vi "NMRvmeCard3.vi"() -> ()   [LabVIEW 2013]
uses:
  <vilib>/Utility/file.llb/Read From Spreadsheet File (DBL).vi
  <vilib>/Analysis/NI_AALBase.lvlib
panel:
  in  "Max":bool=TRUE
  in  "Logoffset (V)":dbl=-5.924000000000002 min=-9.0 max=0.0 step=0.0005 format="%_5g"
  in  "Phase (V)":dbl=6.5 min=0.0 max=9.0 step=0.0005 format="%_5g"
  out "Telnet error out":errorcluster
  in  "Real/Quad Q curve":bool=TRUE
  out "Temperature (C)":dbl(graph)=27.5
  out "+3V supply":dbl=3.245 format="%_4g"
  out "Temp (C)":dbl=27.5 format="%_4g"
  in  "RemovePed":bool=TRUE
  in  "IF / LOG Det":bool
  in  "Q curve file":string="realback213.txt"
  out "File name 2":string="C:\\users\\plm\\Desktop\\rssmt\\realback213.txt"
  in  "AutoTune":bool=TRUE
  out "RF OK":bool=TRUE
  out "Peak area (V-MHz)":sgl=0.028832752 format="%.5f"
  in  "Gauss Fit":bool
  out "NMR Graph + Fit":cluster{cluster{dbl, "Numeric":dbl}[]}[](graph)=[{[{212.6, "Numeric"=-0.048532500000002754}, {212.60999999999999, "Numeric"=-0.03653250000002278}, {212.62, "Numeric"=-0.045792499999980585}, {212.63, "Numeric"=-0.04201250000000012}, {212.64, "Numeric"=-0.04119250000001873}, {212.65, "Numeric"=-0.031632499999979746}, {212.66, "Numeric"=-0.02963249999999795}, {212.67, "Numeric"=-0.03309250000001501}, {212.68, "Numeric"=-0.02891249999997941}, {212.69, "Numeric"=-0.03189249999999605}, {212.7, "Numeric"=-0.022732500000011698}, {212.71, "Numeric"=-0.01753249999997938}, {212.72, "Numeric"=-0.024692499999994646}, {212.73, "Numeric"=-0.01491250000000879}, {212.74, "Numeric"=-0.010992500000022023}, {212.75, "Numeric"=-0.011032499999993586}, {212.76, "Numeric"=0.0010674999999937297}, {212.77, "Numeric"=-0.008192500000018001}, {212.78, "Numeric"=-0.02261249999999287}, {212.79, "Numeric"=-0.024392500000004116}, {212.8, "Numeric"=-0.032232500000014375}, {212.81, "Numeric"=-0.027532499999992573}, {212.82, "Numeric"=-0.02899250000000236}, {212.82999999999998, "Numeric"=-0.024212500000011152}, {212.84, "Numeric"=-0.03769249999999266}, {212.85, "Numeric"=-0.039132500000000986}, {212.85999999999999, "Numeric"=-0.023232500000008306}, {212.87, "Numeric"=-0.016892499999993125}, {212.88, "Numeric"=0.0014875000000000131}, {212.89, "Numeric"=-0.004392500000005847}, {212.9, "Numeric"=0.00376750000000603}, {212.91, "Numeric"=0.008167500000000622}, {212.92, "Numeric"=-0.00019250000000377299}, {212.93, "Numeric"=0.00618750000000479}, {212.94, "Numeric"=0.01090750000000085}, {212.95, "Numeric"=0.03826749999999793}, {212.96, "Numeric"=0.09656750000000316}, {212.97, "Numeric"=0.1705075000000007}, {212.98, "Numeric"=0.3255874999999992}, {212.99, "Numeric"=0.3123074999999988}, {213.0, "Numeric"=0.22976750000000018}, {213.01, "Numeric"=0.20266750000000014}, {213.02, "Numeric"=0.18930750000000116}, {213.03, "Numeric"=0.14968749999999922}, {213.04, "Numeric"=0.1382075000000007}, {213.05, "Numeric"=0.14966750000000317}, {213.06, "Numeric"=0.1471674999999979}, {213.07, "Numeric"=0.16360750000000085}, {213.08, "Numeric"=0.1525875000000048}, {213.09, "Numeric"=0.09930749999999622}, {213.1, "Numeric"=0.06516750000000061}, {213.11, "Numeric"=0.04746750000000602}, {213.12, "Numeric"=0.04960749999999414}, {213.13, "Numeric"=0.0405875}, {213.14000000000001, "Numeric"=0.024907500000006872}, {213.15, "Numeric"=0.013367499999991695}, {213.16, "Numeric"=0.014667499999999018}, {213.17000000000002, "Numeric"=0.029707500000007343}, {213.18, "Numeric"=0.04208749999998884}, {213.19, "Numeric"=0.029407499999997647}, {213.2, "Numeric"=0.038467500000007426}, {213.21, "Numeric"=0.038667499999985616}, {213.22, "Numeric"=0.016007499999995876}, {213.23, "Numeric"=0.023787500000007126}, {213.24, "Numeric"=0.03210750000001941}, {213.25, "Numeric"=0.03386749999999372}, {213.26, "Numeric"=0.015167500000006415}, {213.27, "Numeric"=0.018307500000020214}, {213.28, "Numeric"=0.0113874999999912}, {213.29, "Numeric"=0.021007500000005373}, {213.3, "Numeric"=0.0360675000000206}, {213.31, "Numeric"=0.03156749999998826}, {213.32, "Numeric"=0.03200750000000396}, {213.33, "Numeric"=0.0359875000000206}, {213.34, "Numeric"=0.032307499999984945}, {213.35, "Numeric"=0.03296750000000209}, {213.36, "Numeric"=0.026367500000020253}, {213.37, "Numeric"=0.016907499999981316}, {213.38, "Numeric"=0.011387499999999887}, {213.39000000000001, "Numeric"=0.014307500000019461}, {213.4, "Numeric"=0.018367499999977225}]}]
  in  "Amp of Q curve":dbl=2.800000000000001 min=0.0 max=9.0 step=0.01 format="%_3f"
  in  "Subtract Q curve":bool=TRUE
  in  "Adjust Tune":bool=TRUE
  out "Pedestal Offset":dbl(graph)=0.026662499999999974
  out "Pedestal Difference":dbl(graph)=0.05318500000000375
  out "# Good Spectra":i32=9865
  in  "Quality cuts":bool=TRUE
  out "Pedestal OK":bool=TRUE
  out "Sweep #":i32=122
  out "1st Sweep":bool
  out "ADC volts OK":bool=TRUE
  out "Peak Height Distribution":cluster{"Y":dbl[], "Y":dbl[]}[](graph)=[{"Y"=[0.29554139583333255, 0.2962908541666659, 0.29704031249999924, 0.2977897708333326, 0.2985392291666659, 0.29928868749999926, 0.3000381458333326, 0.3007876041666659, 0.30153706249999923, 0.3022865208333326, 0.3030359791666659, 0.30378543749999926, 0.3045348958333326, 0.3052843541666659, 0.3060338124999992, 0.30678327083333257, 0.3075327291666659, 0.30828218749999925, 0.3090316458333326, 0.30978110416666593, 0.3105305624999992, 0.31128002083333256, 0.3120294791666659, 0.31277893749999924, 0.3135283958333326, 0.3142778541666659, 0.31502731249999927, 0.31577677083333255, 0.3165262291666659, 0.31727568749999924, 0.3180251458333326, 0.3187746041666659, 0.31952406249999926, 0.32027352083333255, 0.3210229791666659, 0.32177243749999923, 0.3225218958333326, 0.3232713541666659, 0.32402081249999926, 0.3247702708333326, 0.3255197291666659, 0.3262691874999992, 0.32701864583333257, 0.3277681041666659, 0.32851756249999925, 0.3292670208333326, 0.33001647916666593, 0.3307659374999992, 0.33151539583333256, 0.3322648541666659, 0.33301431249999924, 0.3337637708333326, 0.3345132291666659, 0.3352626874999992, 0.33601214583333255, 0.3367616041666659, 0.33751106249999924, 0.3382605208333326, 0.3390099791666659, 0.33975943749999926, 0.34050889583333255, 0.3412583541666659, 0.34200781249999923, 0.3427572708333326, 0.3435067291666659, 0.34425618749999926, 0.3450056458333326, 0.3457551041666659, 0.3465045624999992, 0.34725402083333257, 0.3480034791666659, 0.34875293749999925, 0.3495023958333326, 0.3502518541666659, 0.3510013124999992, 0.35175077083333256, 0.3525002291666659, 0.35324968749999924, 0.3539991458333326, 0.3547486041666659, 0.3554980624999992, 0.35624752083333255, 0.3569969791666659, 0.35774643749999924, 0.3584958958333326, 0.3592453541666659, 0.35999481249999926, 0.36074427083333255, 0.3614937291666659, 0.36224318749999923, 0.3629926458333326, 0.3637421041666659, 0.36449156249999926, 0.36524102083333254, 0.3659904791666659, 0.3667399374999992, 0.36748939583333257, 0.3682388541666659, 0.36898831249999925, 0.3697377708333326], "Y"=[10.0, 7.0, 8.0, 10.0, 9.0, 12.0, 15.0, 17.0, 25.0, 21.0, 45.0, 32.0, 38.0, 31.0, 45.0, 39.0, 58.0, 47.0, 54.0, 69.0, 66.0, 80.0, 83.0, 84.0, 100.0, 76.0, 103.0, 100.0, 102.0, 140.0, 106.0, 129.0, 140.0, 149.0, 172.0, 159.0, 139.0, 164.0, 175.0, 192.0, 172.0, 196.0, 176.0, 188.0, 194.0, 191.0, 209.0, 193.0, 182.0, 188.0, 192.0, 215.0, 195.0, 176.0, 186.0, 181.0, 198.0, 183.0, 163.0, 185.0, 179.0, 217.0, 160.0, 144.0, 166.0, 139.0, 140.0, 135.0, 128.0, 129.0, 122.0, 110.0, 95.0, 95.0, 99.0, 87.0, 88.0, 80.0, 75.0, 59.0, 62.0, 64.0, 47.0, 39.0, 56.0, 37.0, 33.0, 37.0, 31.0, 26.0, 23.0, 38.0, 20.0, 16.0, 15.0, 14.0, 12.0, 11.0, 15.0, 8.0]}]
  in  "# of Sweeps":i32=10000
  out "S/N":dbl=23.321076865241377 format="%_3g"
  out "Peak mean (V)":dbl=0.33264146300050557 format="%_4g"
  out "Peak Height":dbl(graph)=0.3255874999999992
  in  "Raw Data":bool=TRUE
  in  "Tank RF":bool=TRUE
  in  "IF Atten (dB)":i8=4 min=0 max=31 step=1
  in  "IFoffset (V)":dbl=6.543044000000001 min=-0.0 max=9.0 step=0.001 format="%.4f"
  in  "Tune  (V)":dbl=1.0950000000000002 min=-0.5 max=5.0 step=0.001 format="%.4f"
  in  "Hi / Lo Gain":bool
  out "Voltage Array":sgl[](array[numeric])=[0.4374, 0.427, 0.3959, 0.3784, 0.3585, 0.3479, 0.3303, 0.3078, 0.2935, 0.2726, 0.2644, 0.2528, 0.2294, 0.2235, 0.2123, 0.1977, 0.1958, 0.1731, 0.1458, 0.1317, 0.1121, 0.1056, 0.0935, 0.0882, 0.0652, 0.0548, 0.0623, 0.0608, 0.0719, 0.0593, 0.0613, 0.0601, 0.0467, 0.0486, 0.0494, 0.0734, 0.1289, 0.2006, 0.354, 0.3396, 0.2565, 0.2294, 0.2166, 0.1781, 0.1683, 0.182, 0.1823, 0.2021, 0.195, 0.1462, 0.1171, 0.105, 0.1133, 0.111, 0.1026, 0.0989, 0.1086, 0.1326, 0.1545, 0.1519, 0.1716, 0.183, 0.1721, 0.1922, 0.2134, 0.2286, 0.2239, 0.2416, 0.2498, 0.2751, 0.3064, 0.3187, 0.3365, 0.3584, 0.3732, 0.3929, 0.4059, 0.4166, 0.4318, 0.456, 0.4819] format="%.4f"
  in  "Invert Polarity":bool=TRUE
  out "Pedestal Diff (V)":sgl=0.053185 format="%.3f"
  out "Peak amp (V)":sgl=0.3255875 format="%.3f"
  in  "Save Data to File":bool
  in  "RF Level (dBm)":dbl min=-10.0 max=10.0 step=0.1 format="%.2f"
  out "SMT error out":errorcluster
  out "Sample RMS (V)":dbl=0.009938271604938272 format="%.4f"
  in  "# Sample/step":i32=80 min=1 max=1000 step=100
  in  "Step Width (MHz)":dbl=0.01 min=0.0 max=1000.0 step=0.0005 format="%.4f"
  in  "Freq Span (MHz)":dbl=0.8 min=0.0 max=3000.0 step=0.1 format="%.3f"
  in  "Center Freq (MHz)":dbl=213.0 min=0.005 max=6000.0 step=0.1 format="%.3f"
  in  "Sweep Mode":u16(ring)=3 items=["Off", "Single", "Auto", "Step"]
  in  "GPIB Addr (28)":refnum<visa-resource-name>="GPIB0::28::INSTR"
  # "E1039 Prototype NMR Control Panel"
  # "Settings"
  # "D\nA\nC"
  # "R\nF\n\nG\nE\nN \n\n+\n\nI\nF"
  # "A\nD\nC"
  # "I\n/\nO"
  # "D\nA\nT\nA\n\nA \nN\nA\nL\nY\nS\nI\nS"
  # "Results"
  # "A\nv\ne\nr\na\ng\ne"
  # "S\nw\ne\ne\np"
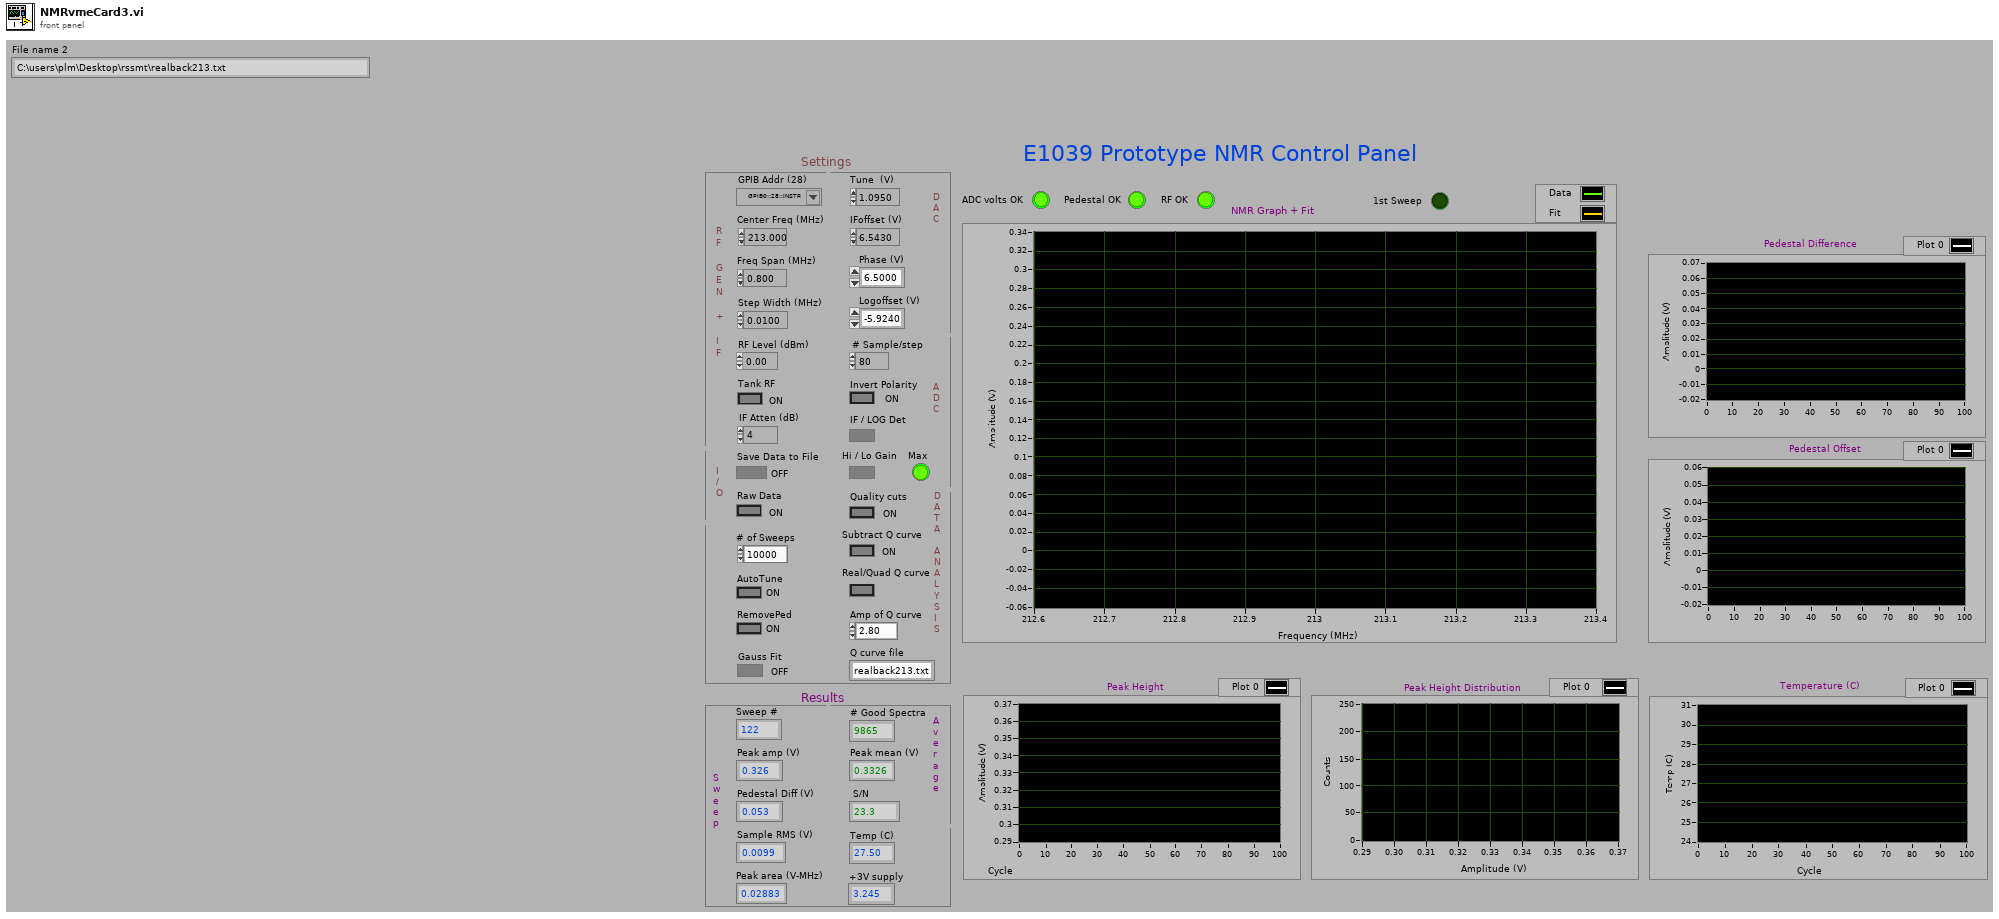
[diagram p1: front panel]
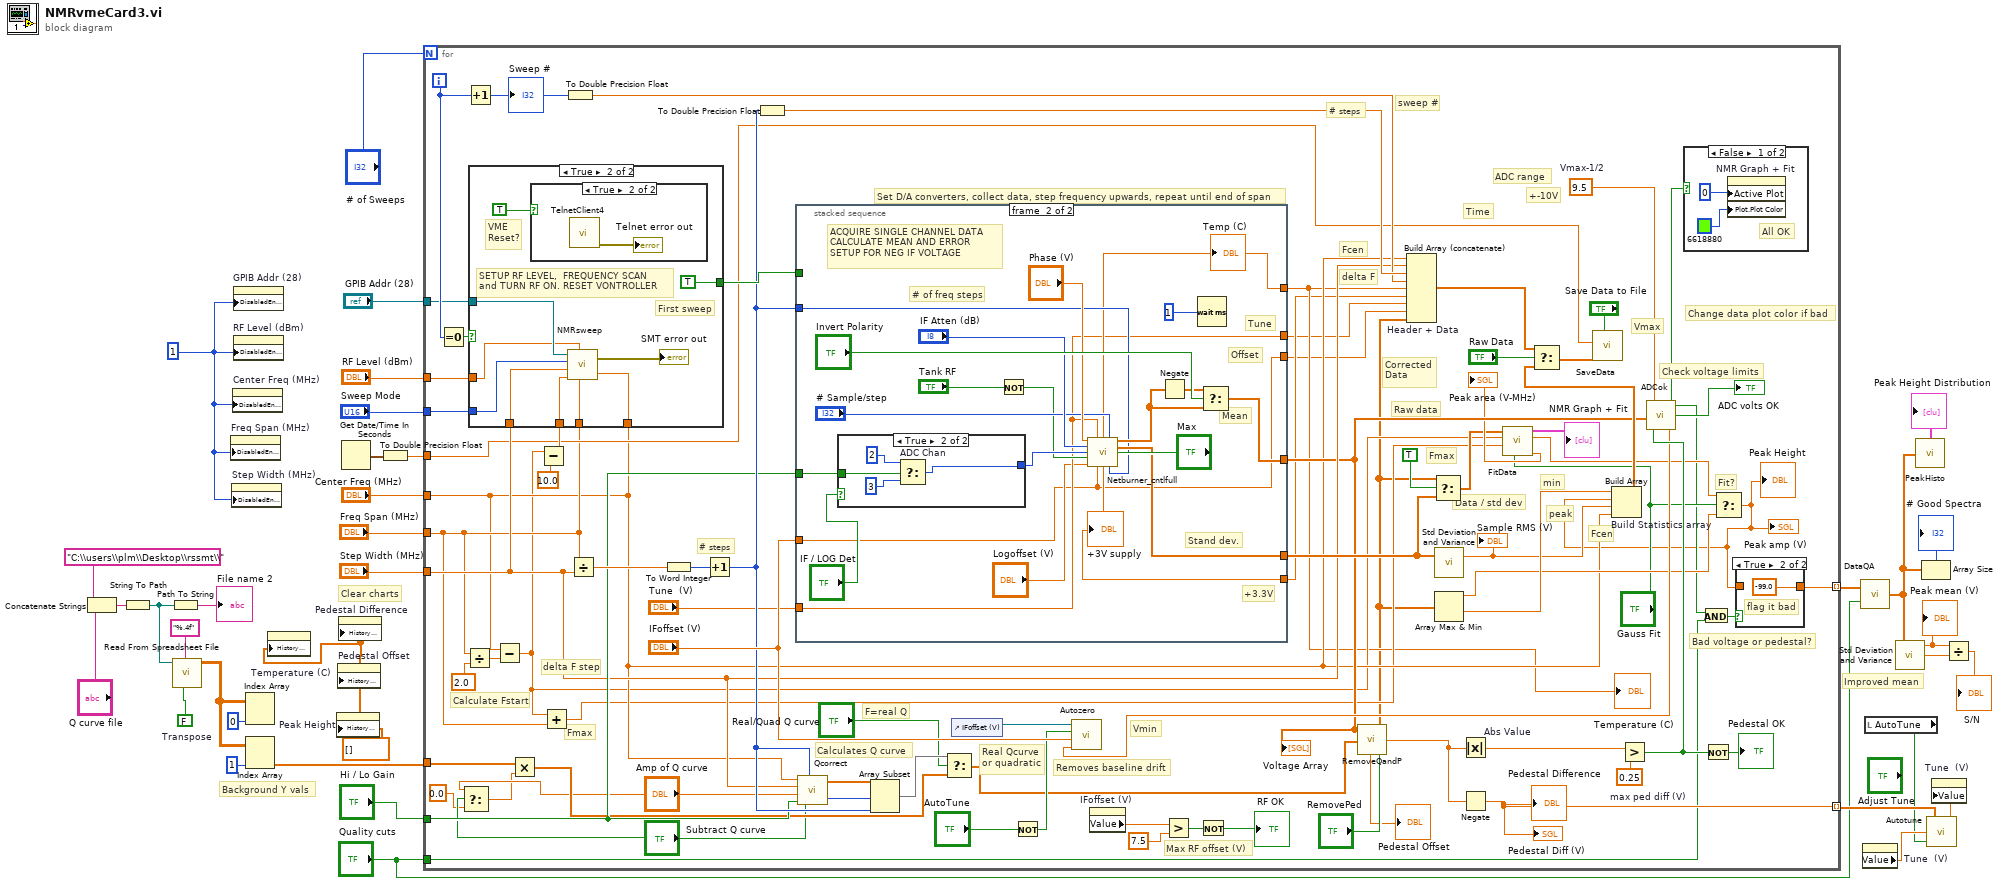
[diagram p0: block diagram]
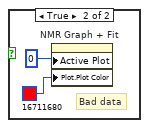
[diagram p2: hidden frame]
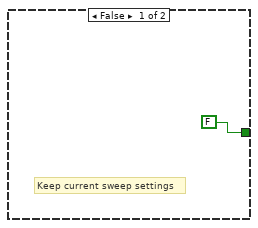
[diagram p4: hidden frame]
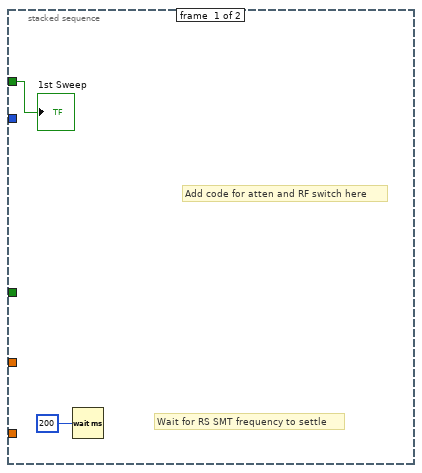
[diagram p6: hidden frame]
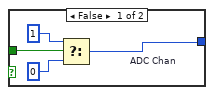
[diagram p7: hidden frame]
diagram:
  w2 = 1
  w14 = FALSE  # Transpose
  w6 = dbl[] []
  # "Background Y vals"
  # "Clear charts"
  # "Improved mean"
  n1 = Concatenate Strings "Concatenate Strings"("C:\\users\\plm\\Desktop\\rssmt\\", "Q curve file") -> (w17:string)
  n2 = String To Path(string=w17) -> (path=w13:path)
  n3 = Path To String(path=w13) -> (string=→"File name 2":string)
  n4 = call-poly <vilib>:"Read From Spreadsheet File.vi"("transpose (no:F)"=w14, "format (%.3f)"="%.4f", "file path (dialog if empty)"=w13) -> ("all rows"=w12:dbl[][])  [unwired: 4 in, 4 out]
  n5 = property on="Freq Span (MHz)" class="DigNum (strict)"("DisabledEnum"=w2) -> ()  [unwired: 2 in, 2 out]
  n6 = property on="Step Width (MHz)" class="DigNum (strict)"("DisabledEnum"=w2) -> ()  [unwired: 2 in, 2 out]
  n7 = property on="Center Freq (MHz)" class="DigNum (strict)"("DisabledEnum"=w2) -> ()  [unwired: 2 in, 2 out]
  n8 = property on="GPIB Addr (28)" class="VISAName"("DisabledEnum"=w2) -> ()  [unwired: 2 in, 2 out]
  n9 = property on="RF Level (dBm)" class="DigNum (strict)"("DisabledEnum"=w2) -> ()  [unwired: 2 in, 2 out]
  n10 = Index Array "Index Array"(array=w12, index (col)=0) -> ()  [unwired: 1 in, 1 out]
  n11 = Index Array(array=w12, index (col)=1) -> (element=w7:dbl[])  [unwired: 1 in]
  n12 = property on="Temperature (C)" class="WFChart (strict)"("History Data"=w6) -> ()  [unwired: 2 in, 2 out]
  n13 = property on="Peak Height" class="WFChart (strict)"("History Data"=w6) -> ()  [unwired: 2 in, 2 out]
  n14 = property on="Pedestal Offset" class="WFChart (strict)"("History Data"=w6) -> ()  [unwired: 2 in, 2 out]
  n15 = property on="Pedestal Difference" class="WFChart (strict)"("History Data"=w6) -> ()  [unwired: 2 in, 2 out]
  n16 = Get Date/Time In Seconds() -> (seconds since 1Jan1904=w19:timestamp)
  n17 = To Double Precision Float(number=w19) -> (double precision float=w18:dbl)
  n18 = for {
    N: "# of Sweeps" -> [_]
    tunnel: [w99] -> w33 mode=indexing
    tunnel: "Quality cuts" -> [w77]
    tunnel: [w83] -> w30 mode=indexing
    tunnel: "Center Freq (MHz)" -> [w64]
    tunnel: "Freq Span (MHz)" -> [w70]
    tunnel: "Step Width (MHz)" -> [w76]
    tunnel: "Sweep Mode" -> [w87]
    tunnel: "Hi / Lo Gain" -> [w86]
    tunnel: "GPIB Addr (28)" -> [w85]
    tunnel: "RF Level (dBm)" -> [w84]
    tunnel: w18 -> [w71]
    tunnel: w7 -> [w49]
    i -> [w97]
    w81 = 9.5  # Vmax-1/2
    w100 = 0.25  # max ped diff (V)
    # "F=real Q"
    # "Real Qcurve\nor quadratic"
    # "+-10V"
    # "Vmax"
    # "Change data plot color if bad"
    # "Max RF offset (V)"
    # "Fmax"
    # "Fit?"
    # "Fmax"
    # "Time"
    # "Vmin"
    # "min"
    # "peak"
    # "Raw data"
    # "Corrected\nData"
    # "Fcen"
    # "delta F"
    # "# steps"
    # "ADC range"
    # "sweep #"
    # "Fcen"
    # "Set D/A converters, collect data, step frequency upwards, repeat until end of span"
    # "Calculates Q curve"
    # "Removes baseline drift"
    # "Bad voltage or pedestal?"
    # "Check voltage limits"
    # "Data / std dev"
    # "# steps"
    # "Calculate Fstart"
    # "delta F step"
    n19 = Equal To 0?(x=w97) -> (x = 0?=w102:bool)
    n20 = Select(t="Amp of Q curve", s="Subtract Q curve", f=0.0) -> (s? t:f=w44:dbl)
    n21 = Divide(x=w70, y=sgl 2.0) -> (x/y=w113:dbl)
    n22 = Increment(x=w97) -> (x+1=w88:i32)
    "Sweep #" <- w88
    n23 = Subtract(x=w64, y=w113) -> (x-y=w59:dbl)
    n24 = Multiply(x=w49, y=w44) -> (x*y=w48:dbl[])
    n25 = Subtract(x=w59, y=10.0) -> (x-y=w111:dbl)
    n26 = case shown="True" w102 {
      tunnel: w111 -> [_ w132]
      tunnel: w76 -> [_ w130]
      tunnel: w64 -> [_ w129]
      tunnel: w70 -> [_ w131]
      tunnel: [FALSE TRUE] -> w101
      tunnel: w87 -> [_ w126]
      tunnel: w85 -> [_ w125]
      tunnel: w84 -> [_ w124]
      frame False {
        # "Keep current sweep settings"
      }
      frame True {
        # "VME\nReset?"
        # "First sweep"
        # "SETUP RF LEVEL,  FREQUENCY SCAN\nand TURN RF ON. RESET VONTROLLER"
        n27 = case shown="True" TRUE {
          frame False {
          }
          frame True {
            n28 = call "TelnetClient4.vi"() -> ("Telnet error"=→"Telnet error out":errorcluster)  [unwired: 4 in, 3 out]
          }
        }
        n29 = call "NMRsweep.vi"("Center Freq (MHz)"=w129, "Freq Span (MHz)"=w131, "RF Level (dBm)"=w124, "Foffset (MHz)"=w132, "Step Width (MHz)"=w130, "Sweep Mode"=w126, "GPIB Addr (28)"=w125) -> ("error out"=→"SMT error out":errorcluster)
      }
    }
    n30 = Add(x=w59, y=w70) -> (x+y=w58:dbl)
    n31 = To Double Precision Float(number=w88) -> (double precision float=w89:dbl)
    n32 = Divide(x=w70, y=w76) -> (x/y=w115:dbl)
    n33 = To Word Integer(number=w115) -> (16bit integer=w112:i16)
    n34 = Increment(x=w112) -> (x+1=w91:i16)
    n35 = To Double Precision Float(number=w91) -> (double precision float=w90:dbl)
    n36 = stacked-sequence {
      tunnel: [_ w146] -> w105
      tunnel: [_ w154] -> w74
      tunnel: w91 -> [_ w143]
      tunnel: "IFoffset (V)" -> [_ w136]
      tunnel: w86 -> [_ w152]
      tunnel: w101 -> [w134 _]
      tunnel: "Tune  (V)" -> [_ w138]
      tunnel: [_ w142] -> w40
      tunnel: [_ w139] -> w39
      tunnel: [_ w138] -> w37
      tunnel: [_ w136] -> w36
      frame #0 {
        # "Add code for atten and RF switch here"
        # "Wait for RS SMT frequency to settle"
        n37 = Wait (ms)(milliseconds to wait=200) -> ()  [unwired: 1 out]
        "1st Sweep" <- w134
      }
      frame #1 {
        # "+3.3V"
        # "Offset"
        # "Tune"
        # "Stand dev."
        # "Mean"
        # "ACQUIRE SINGLE CHANNEL DATA\nCALCULATE MEAN AND ERROR\nSETUP FOR NEG IF VOLTAGE"
        # "# of freq steps"
        n38 = case shown="True" "IF / LOG Det" {
          tunnel: w152 -> [w160 w161]
          tunnel: [w157 w162] -> w145
          frame False {
            n39 = Select "ADC Chan"(t=1, s=w160, f=0) -> (s? t:f=w157:i32)
          }
          frame True {
            n40 = Select "ADC Chan"(t=2, s=w161, f=3) -> (s? t:f=w162:i32)
          }
        }
        n41 = Not(x="Tank RF") -> (.not. x?=w141:bool)
        n42 = call "Netburner_cntlfull.vi"("Phase Volt"="Phase (V)", "Tune Volt"=w138, "# Data"="# Sample/step", "IF Atten (dB)"="IF Atten (dB)", "NMR ADC"=w145, "Hi Gain"="Max", "Tank RF"=w141, "LogOff Volt"="Logoffset (V)", "IFOff Volt"=w136, "# f steps"=w143) -> ("Temp (C)"=w142:dbl, "ADC value"=w147:dbl[], "ADC error"=w146:dbl[], "Volts"=w139:dbl)  [unwired: 2 out]
        "Temp (C)" <- w142
        "+3V supply" <- w139
        n43 = Negate(x=w147) -> (-x=w153:dbl[])
        n44 = Wait (ms)(milliseconds to wait=1) -> ()  [unwired: 1 out]
        n45 = Select(t=w153, s="Invert Polarity", f=w147) -> (s? t:f=w154:dbl[])
      }
    }
    "Voltage Array" <- w74
    "Temperature (C)" <- w40
    n46 = call "Qcorrect.vi"("Subtract Q curve"="Subtract Q curve", "Nstep"=w91, "IF or Log"=w86, "Amp of Q curve"="Amp of Q curve", "Step Width (MHz)"=w76, "Center Freq (MHz)"=w64) -> ("Start"=w106:i32, "Array"=w107:dbl[])
    n47 = Array Subset "Array Subset"(array=w107, index=w106, length=w91) -> (w52:dbl[])
    n48 = Select(t=w52, s="Real/Quad Q curve", f=w48) -> (s? t:f=w51:dbl[])
    n49 = control-ref of="IFoffset (V)"() -> (w80:refnum<vi>)
    n50 = Not(x="AutoTune") -> (.not. x?=w53:bool)
    n51 = property on="IFoffset (V)" class="DigNum (strict)"() -> ("Value"=w68:dbl)  [unwired: 2 in, 2 out]
    n52 = Greater?(x=w68, y=7.5) -> (0:w66:bool)
    n53 = Not(x=w66) -> (.not. x?=→"RF OK":bool)
    n54 = call "RemoveQandP.vi"("Subtract Ped?"="RemovePed", "Qcurve"=w51, "Raw data"=w74) -> ("Ped L-R"=w93:dbl, "Corrected data"=w38:dbl[], "Ped Offfset"=→"Pedestal Offset":dbl)
    n55 = Build Array (concatenate) "Header + Data"(w64, w76, w90, w89, w40, w39, w37, w36, w38) -> (w92:dbl[])
    n56 = Select(t=w38, s=TRUE, f=w105) -> (s? t:f=w60:dbl[])
    n57 = call <vilib>:"Std Deviation and Variance.vi"("X"=w105) -> ("mean"=w75:dbl)  [unwired: 1 in, 2 out]
    "Sample RMS (V)" <- w75
    n58 = Array Max & Min(array=w38) -> (max value=w69:dbl, min value=w104:dbl)  [unwired: 2 out]
    n59 = Absolute Value "Abs Value"(x=w93) -> (abs(x)=w95:dbl)
    n60 = Negate(x=w93) -> (-x=w83:dbl)
    "Pedestal Diff (V)" <- w83
    "Pedestal Difference" <- w83
    n61 = call "FitData.vi"("Fit?"="Gauss Fit", "Fmax"=w58, "Fmin"=w59, "Yarray"=w60) -> ("Peak Area (V-MHz)"=→"Peak area (V-MHz)":dbl, "Amplitude (V)"=w62:dbl, "NMR Graph + Fit"=→"NMR Graph + Fit":cluster{cluster{dbl, "Numeric":dbl}[]}[])  [unwired: 2 out]
    n62 = Greater?(x=w95, y=w100) -> (0:w82:bool)
    n63 = call "ADCok.vi"("PedOK"=w82, "Array"=w74, "Vmax-1/2"=w81) -> ("Vmin"=w79:dbl, "ADC voltages OK"=→"ADC volts OK":bool, "Allok"=w56:bool)
    n64 = call "Autozero.vi"("Vmin (V)"=w79, "IFoffset (V)"="IFoffset (V)", "IF or Log"=w53, "reference"=w80) -> ()
    n65 = case shown="False" w56 {
      frame False {
        # "All OK"
        n66 = property on="NMR Graph + Fit" class="XYGraph (strict)"("Active Plot"=0, "Plot.Plot Color"=u32 6618880) -> ()  [unwired: 2 in, 2 out]
      }
      frame True {
        # "Bad data"
        n67 = property on="NMR Graph + Fit" class="XYGraph (strict)"("Active Plot"=0, "Plot.Plot Color"=u32 16711680) -> ()  [unwired: 2 in, 2 out]
      }
    }
    n68 = And(x=w56, y=w77) -> (x .and. y?=w96:bool)
    n69 = Not(x=w82) -> (.not. x?=→"Pedestal OK":bool)
    n70 = Select(t=w62, s="Gauss Fit", f=w69) -> (s? t:f=w55:dbl)
    "Peak amp (V)" <- w55
    "Peak Height" <- w55
    n71 = Build Array "Build Statistics array"(w104, w55, w75, w64) -> (w110:dbl[])
    n72 = Select(t=w92, s="Raw Data", f=w110) -> (s? t:f=w72:dbl[])
    n73 = call "SaveData.vi"("Array"=w72, "Save Data to File"="Save Data to File", "Ext time (sec)"=w71) -> ()  [unwired: 1 out]
    n74 = case shown="True" w96 {
      tunnel: [w120 -99.0] -> w99
      tunnel: w55 -> [w120 _]
      frame False {
        # "Data OK"
      }
      frame True {
        # "flag it bad"
      }
    }
  }
  n75 = call "DataQA.vi"("Quality cuts"="Quality cuts", "Data In"=w33) -> ("Data Out"=w32:dbl[])
  n76 = property on="Tune  (V)" class="DigNum (strict)"() -> ("Value"=w22:dbl)  [unwired: 2 in, 2 out]
  n77 = local read "AutoTune"() -> (w1:bool)
  n78 = call <vilib>:"Std Deviation and Variance.vi"("X"=w32) -> ("mean"=w5:dbl, "standard deviation"=w4:dbl)  [unwired: 1 in, 1 out]
  "Peak mean (V)" <- w5
  n79 = call "PeakHisto.vi"("Data Out"=w32) -> ("XY Graph"=→"Peak Height Distribution":cluster{"Y":dbl[], "Y":dbl[]}[])
  n80 = Array Size(array=w32) -> (size(s)=→"# Good Spectra":i32)
  n81 = call "Autotune.vi"("Adjust Tune"=w1, "Tune Vin"=w22, "Pedestal Diff"=w30) -> ("Tune Vout"=w21:dbl)
  n82 = property on="Tune  (V)" class="DigNum (strict)"("Value"=w21) -> ()  [unwired: 2 in, 2 out]
  n83 = Divide(x=w5, y=w4) -> (x/y=→"S/N":dbl)
